vi "Get Projectile Atributes.vi"(2 "projectile":refnum<vi>) -> (0 "projectileAttribs":T1)   [LabVIEW 2010]
panel:
  out "error out":errorcluster
  in  "error IN":errorcluster
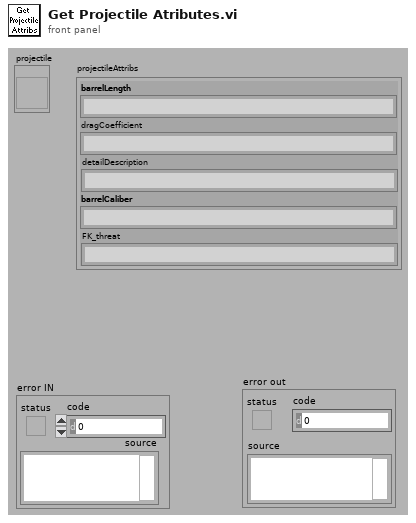
[diagram p1: front panel]
types:
  T1 = cluster{"barrelLength":string, "dragCoefficient":string, "detailDescription":string, "barrelCaliber":string, "FK_threat":string}
  T2 = cluster{"[0]":string, "[1]":string, "[2]":string, "[3]":string, "[4]":string}
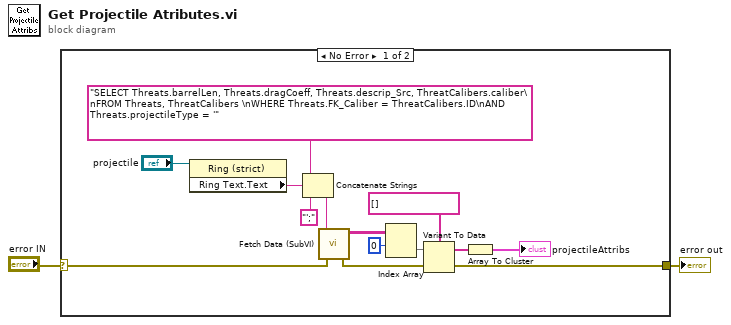
[diagram p0: block diagram]
diagram:
  n1 = case shown="No Error" "error IN" {
    selector: "error IN" -> [w5 w17]
    tunnel: [w3 w17] -> w1
    frame No Error {
      n2 = property on="Property Node" class="Ring (strict)"(reference="projectile") -> ("Ring Text.Text"=w14:string)  [unwired: 1 in, 2 out]
      n3 = Concatenate Strings("SELECT Threats.barrelLen, Threats.dragCoeff, Threats.descrip_Src, ThreatCalibers.caliber\nFROM Threats, ThreatCalibers \nWHERE Threats.FK_Caliber = ThreatCalibers.ID\nAND Threats.projectileType = '", w14, "';" ("string")) -> (w6:string)
      n4 = call "Fetch Data (SubVI).vi"("error IN"=w5, "query string"=w6) -> ("error OUT"=w4:errorcluster, "recordset data"=w16:string[][])  [unwired: 4 out]
      n5 = Index Array(array=w16, index (row)=0 ("disabled index (col)")) -> (element=w10:string[])  [unwired: 1 in]
      n6 = Variant To Data(error in=w4, Variant=w10, type=string[] []) -> (error out=w3:errorcluster, data=w8:string[])
      n7 = Array To Cluster(array=w8) -> (cluster=→"projectileAttribs":T2)
    }
    frame Error {
    }
  }
  "error out" <- w1
